vi "FPGA_main_simplified.vi"() -> ()   [LabVIEW 2024]
uses:
  <vilib>/Platform/TimedLoop/XDataNode/timing_clust.ctl
  <vilib>/Platform/TimedLoop/XDataNode/nitl_modes.ctl
  <vilib>/Platform/TimedLoop/XDataNode/wakeup.ctl
  <vilib>/LabVIEW Targets/FPGA/cRIO/shared/nicrio_ModuleControls/nicrio_cRIO-9775_ContinuousDataRates4ChansRing.ctl
  <vilib>/rvi/Emulation/niFpgaGetClockAttributes.vi
  <vilib>/rvi/Emulation/niFpgaSctlEmulationGetInTimedLoop.vi
  <vilib>/rvi/Emulation/niFpgaEmulationReportErrorSimple.vi
  <vilib>/rvi/Emulation/niFpgaProcessEmulError.vi
  <vilib>/rvi/Emulation/niFpgaCriticalErrorInLSC.vi
  <vilib>/rvi/eio/common/nirviEmuTemplateMethod_errors.vi
  <vilib>/rvi/eio/common/nirviEmuTemplatePropertySet_errors.vi
  <vilib>/eio/utilities/niEioResolveVilibRelativePath.vi
  <vilib>/rvi/interface/RandomDataEmulation/niFpgaRandomDataHandleErrors.vi
  <vilib>/platform/TimedLoop/XDataNode/XDataNode.xnode
  <vilib>/eio/EIONode/EIONode.xnode
  <vilib>/eio/EIOMethodNode/EIOMethodNode.xnode
  <vilib>/eio/EIOPropertyNode/EIOPropertyNode.xnode
  <vilib>/rvi/DataTransferAndStorage/Container/XNode/niFpgaContainer.xnode
  <vilib>/rvi/interface/RandomDataEmulation/nirviRandomDataFpgaReadWriteTemplate.vi
  <vilib>/Platform/TimedLoop/XDataNode/XDNodeRunTimeDep.lvlib
  <vilib>/rvi/eio/common/nirviEmuTemplatePropertyGet_errors.vi
  <vilib>/rvi/eio/common/nirviEmuTemplatePropertyGet_noerrors.vi
  <vilib>/rvi/eio/common/nirviEmuTemplatePropertySet_noerrors.vi
panel:
  out "FPGA routine\nrunning":bool
  in  "Pulse\nWidth":u32 caption="Pulse width(uSec)"
  in  "Pulse\nPeriod":u32 caption="Period(uSec)"
  in  "Stop Routine":bool
  in  "DIO3":bool
  in  "DIO2":bool
  in  "DIO1":bool
  in  "DIO0":bool
  out "Rebinned Counts":i32
  in  "Binning Time (ticks)":i32=1200000
  out "Counts":u8
  out "FPGA Error":errorcluster
  out "Finished":bool
  in  "Stop":bool
  out "Module Underflow":bool
  out "DMA FIFO Full":bool
  out "Actual Loop Period (ticks)":u32=40
  out "First Read":bool
  in  "Type Counter":enum16{"Falling Edge", "Rising Edge"}(ring)
  # "Photon counting. Single cycle time loop"
  # "User Control of digital output"
  # "Thresholding"
  # "Pulsing DIO 0 (Pulse width should be shorter than\n period)"
  # "Binning and streaming binned Total Count"
  # "Streaming Analog Input Data"
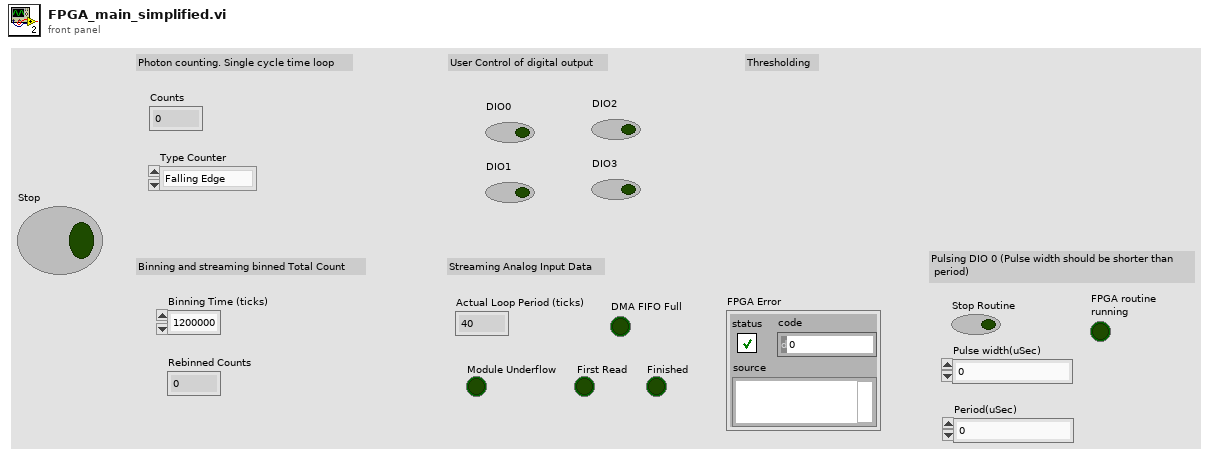
[diagram p1: front panel]
types:
  T1 = typedef "nicrio_cRIO-9775_ContinuousDataRates4ChansRing.ctl" = u16
  T2 = typedef "XDNodeRunTimeDep.lvlib/timing_clust.ctl" = cluster{"Expected End [f-1]":u64, "Actual End [f-1]":u64, "Finished Late? [f-1]":bool, "Expected End [i-1]":u64, "Actual End [i-1]":u64, "Finished Late? [i-1]":bool, "Expected Start [i]":u64, "Actual Start [i]":u64, "Expected Start [f]":u64, "Actual Start [f]":u64, "Source Name":string, "Structure Name":string, "Period":i64, "Deadline":i64, "Offset":i64, "Start":i64, "Priority":i32, "Timeout":i32, "Mode":T3, "Wakeup Reason":T4, "Error":errorcluster, "Source Type":string, "Secondary Source Type":string, "Global End Time":u64, "Global Start Time":u64, "Frame Duration":u64, "Iteration Duration":u64, "Assigned CPU":i32, "I/O Scan Engine Mode":u32}
  T3 = typedef "XDNodeRunTimeDep.lvlib/nitl_modes.ctl" = enum32{"No Change", "Process missed periods, maintain original phase", "Discard missed periods, maintain original phase", "Process missed periods, ignore original phase", "Discard missed periods, ignore original phase"}
  T4 = typedef "XDNodeRunTimeDep.lvlib/wakeup.ctl" = enum32{"Normal", "Aborted", "Asynchronous wakeup", "Timing source error", "Timed loop error", "Timeout"}
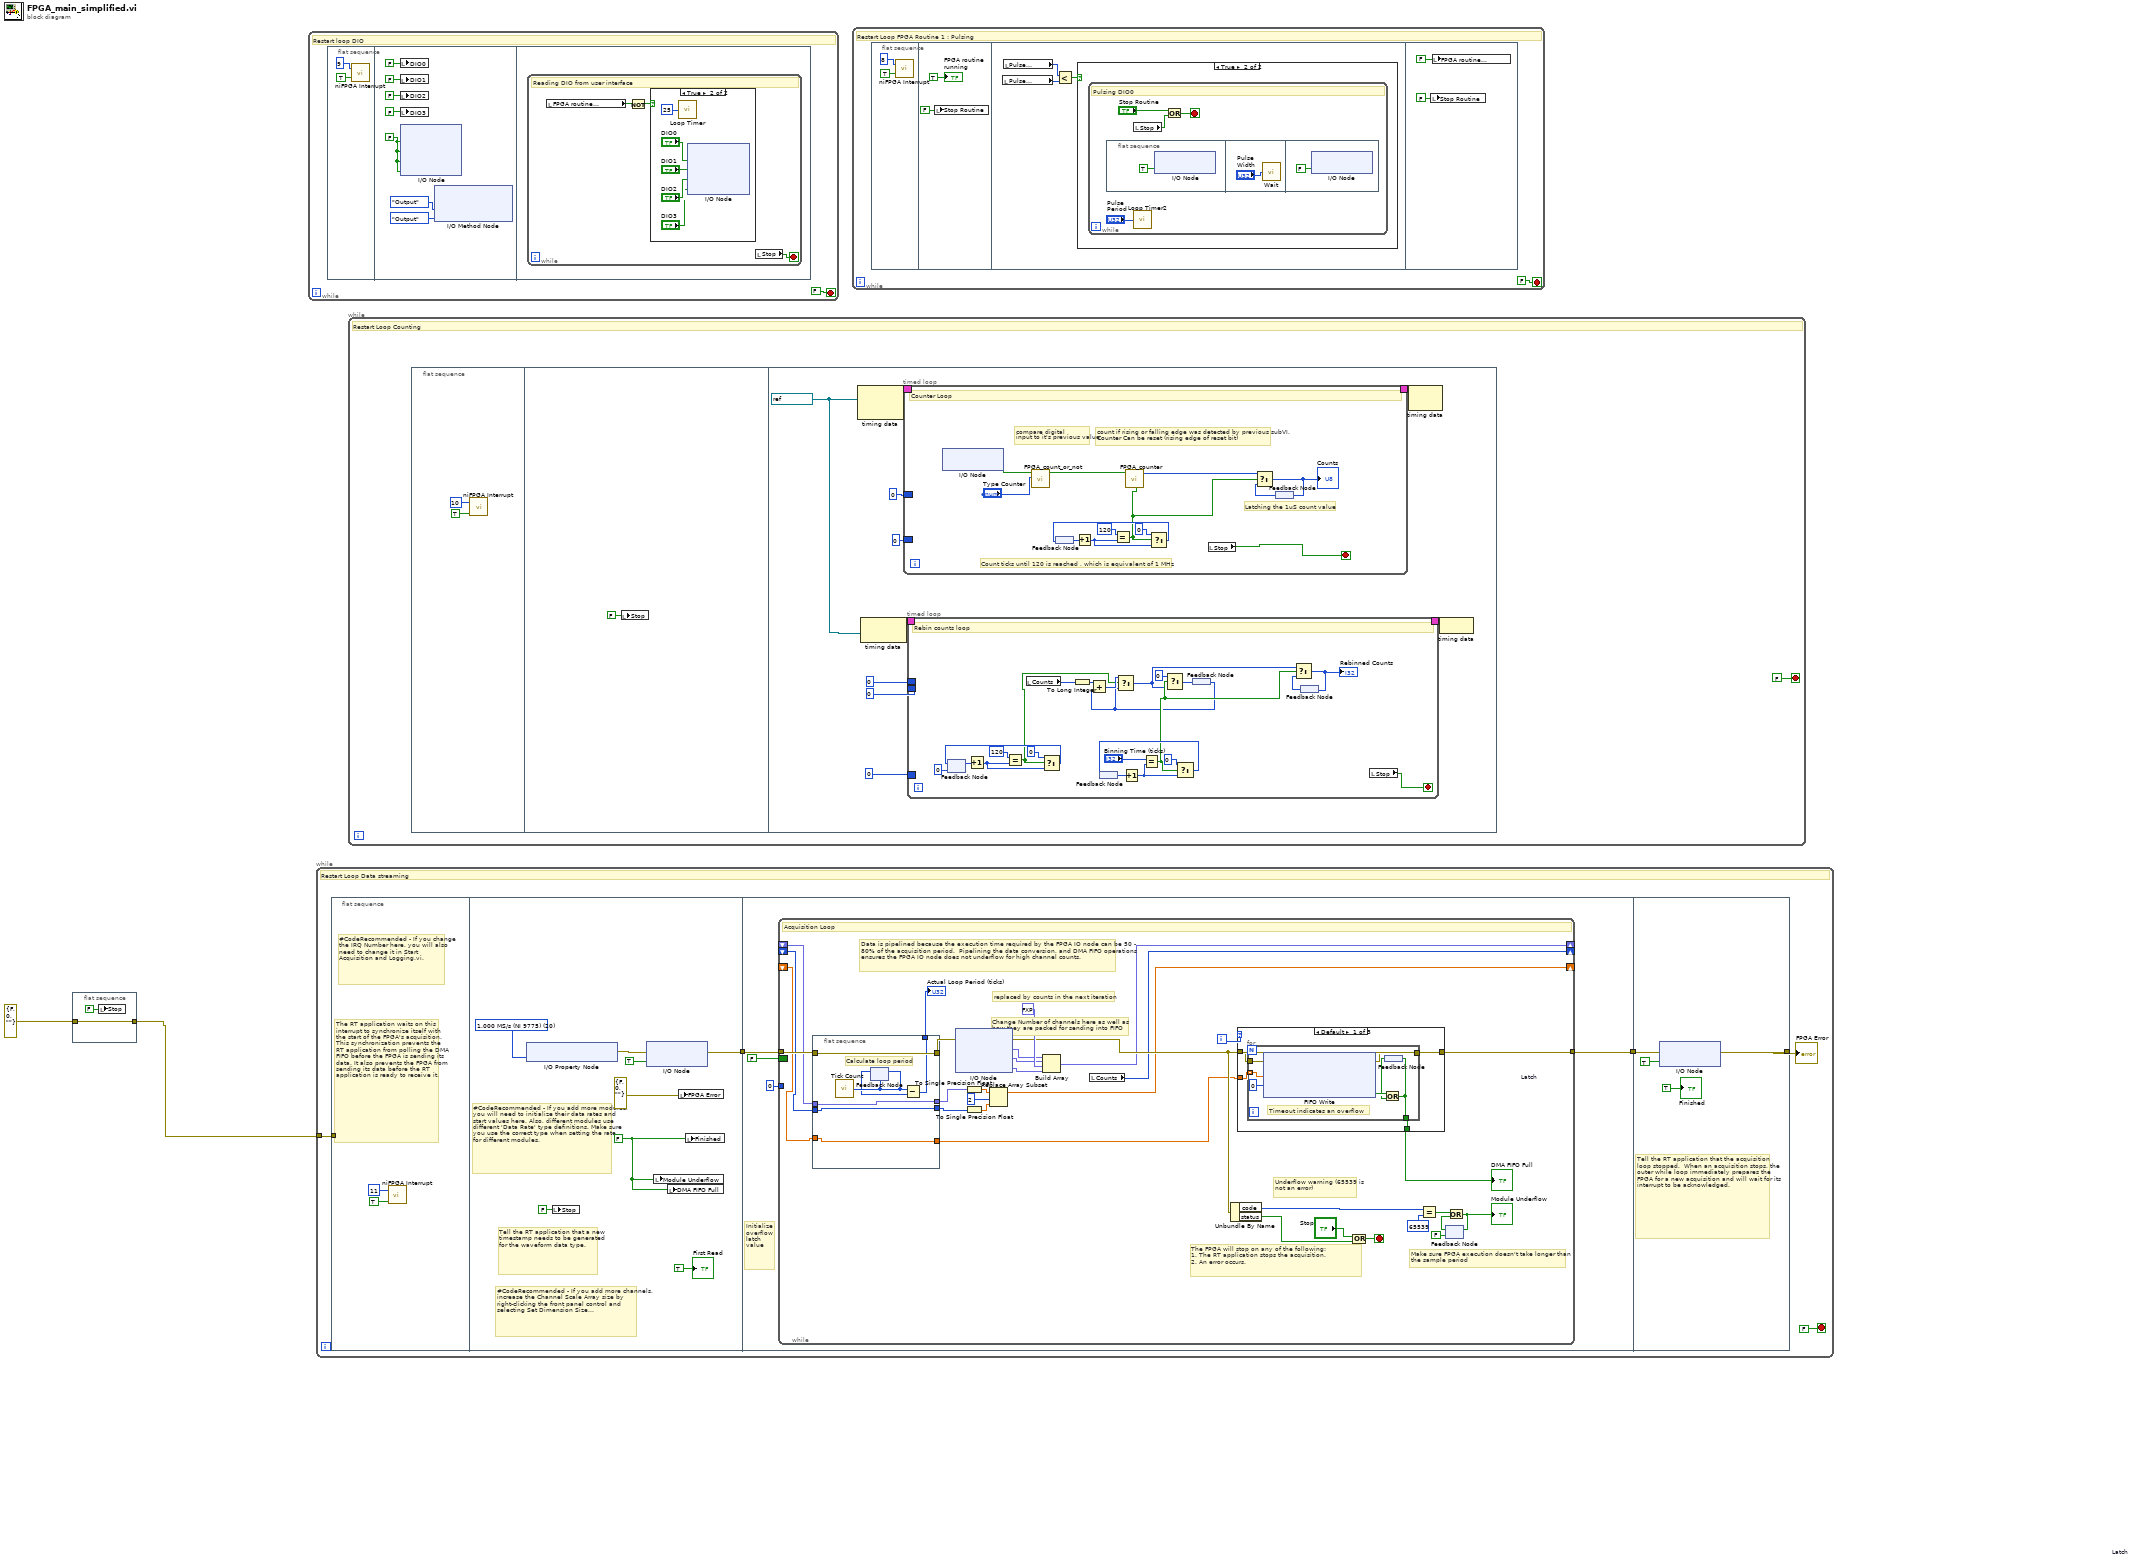
[diagram p0: block diagram]
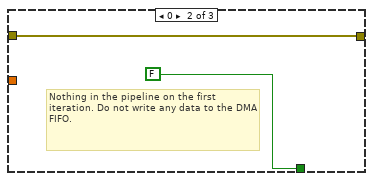
[diagram p4: hidden frame]
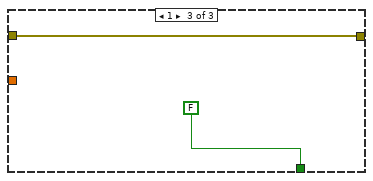
[diagram p5: hidden frame]
diagram:
  n1 = flat-sequence {
    tunnel: errorcluster {"status"=FALSE, "code"=0, "source"=""} ("Error") -> [w3]
    tunnel: [w3] -> w1
    frame #0 {
      n2 = local write "Stop"(FALSE ("stop")) -> ()
    }
  }
  n3 = while {
    stop <- FALSE stop-if-true
    # "Restart loop DIO"
    n4 = flat-sequence {
      frame #0 {
        n5 = call <vilib>:"niFPGA Interrupt.vi"("Wait Until Cleared (F)"=TRUE ("Wait Until Cleared"), "IRQ Number (0)"=u8 9 ("IRQ Number")) -> ()  [unwired: 1 in]
      }
      frame #1 {
        w10 = FALSE ("Mod3/DIO0")
        n6 = local write "DIO0"(FALSE ("DIO0")) -> ()
        n7 = local write "DIO1"(FALSE ("DIO1")) -> ()
        n8 = local write "DIO2"(FALSE ("DIO2")) -> ()
        n9 = local write "DIO3"(FALSE ("DIO3")) -> ()
        n10 = xnode "I/O Node"("Mod3/DIO0"=w10, "Mod3/DIO1"=w10, "Mod3/DIO2"=w10, "Mod3/DIO3"=w10) -> ()  [unwired: 4 in, 4 out]
        n11 = xnode "I/O Method Node"("DIO 7:4"=enum8{"No Change", "Input", "Output"}."Output", "DIO 3:0"=enum8{"No Change", "Input", "Output"}."Output") -> ()  [unwired: 1 in, 1 out]
      }
      frame #2 {
        n12 = while {
          stop <- w17 stop-if-true
          # "Reading DIO from user interface"
          n13 = local read "FPGA routine\nrunning"() -> (w16:bool)
          n14 = Not(x=w16) -> (.not. x?=w15:bool)
          n15 = case shown="True" w15 {
            frame False {
            }
            frame True {
              n16 = call "Loop Timer"("Count(mSec)"=u8 25) -> ()  [unwired: 1 out]
              n17 = xnode "I/O Node"("Mod3/DIO0"="DIO0", "Mod3/DIO1"="DIO1", "Mod3/DIO2"="DIO2", "Mod3/DIO3"="DIO3") -> ()  [unwired: 4 in, 4 out]
            }
          }
          n18 = local read "Stop"() -> (w17:bool)
        }
      }
    }
  }
  n19 = while {
    tunnel: w1 -> [w23]
    stop <- FALSE stop-if-true
    # "Restart Loop Data streaming"
    n20 = flat-sequence {
      tunnel: w23 -> [_]
      tunnel: [w37] -> w26
      tunnel: w26 -> [w39]
      tunnel: [w38] -> w25
      tunnel: w25 -> [w97]
      tunnel: [w96] -> w24
      frame #0 {
        # "#CodeRecommended - If you change the IRQ Number here, you will also need to change it in Start Acquisition and Logging.vi."
        # "The RT application waits on this interrupt to synchronize itself with the start of the FPGA's acquisition.  This synchronization prevents the RT application from polling the DMA FIFO before the FPGA is sending its data. It also prevents the FPGA from sending its data before the RT application is ready to receive it."
        n21 = call <vilib>:"niFPGA Interrupt.vi"("Wait Until Cleared (F)"=TRUE ("Wait Until Cleared"), "IRQ Number (0)"=u8 11 ("IRQ Number")) -> ()  [unwired: 1 in]
      }
      frame #1 {
        w31 = T1 20 items=["1.000 MS/s (NI 9775)"=20, "833.333 KS/s (NI 9775)"=24, "714.286 KS/s (NI 9775)"=28, "625.000 KS/s (NI 9775)"=32, "555.556 KS/s (NI 9775)"=36, "500.000 KS/s (NI 9775)"=40, "454.545 KS/s (NI 9775)"=44, "416.667 KS/s (NI 9775)"=48, "384.615 KS/s (NI 9775)"=52, "357.143 KS/s (NI 9775)"=56, "333.333 KS/s (NI 9775)"=60, "312.500 KS/s (NI 9775)"=64, "294.118 KS/s (NI 9775)"=68, "277.778 KS/s (NI 9775)"=72, "263.158 KS/s (NI 9775)"=76, "250.000 KS/s (NI 9775)"=80, "238.095 KS/s (NI 9775)"=84, "227.273 KS/s (NI 9775)"=88, "217.391 KS/s (NI 9775)"=92, "208.333 KS/s (NI 9775)"=96, "200.000 KS/s (NI 9775)"=100, "192.308 KS/s (NI 9775)"=104, "185.185 KS/s (NI 9775)"=108, "178.571 KS/s (NI 9775)"=112, "172.414 KS/s (NI 9775)"=116, "166.667 KS/s (NI 9775)"=120, "161.290 KS/s (NI 9775)"=124, "156.250 KS/s (NI 9775)"=128, "151.515 KS/s (NI 9775)"=132, "147.059 KS/s (NI 9775)"=136, "142.857 KS/s (NI 9775)"=140, "138.889 KS/s (NI 9775)"=144, "135.135 KS/s (NI 9775)"=148, "131.579 KS/s (NI 9775)"=152, "128.205 KS/s (NI 9775)"=156, "125.000 KS/s (NI 9775)"=160, "121.951 KS/s (NI 9775)"=164, "119.048 KS/s (NI 9775)"=168, "116.279 KS/s (NI 9775)"=172, "113.636 KS/s (NI 9775)"=176, "111.111 KS/s (NI 9775)"=180, "108.696 KS/s (NI 9775)"=184, "106.383 KS/s (NI 9775)"=188, "104.167 KS/s (NI 9775)"=192, "102.041 KS/s (NI 9775)"=196, "100.000 KS/s (NI 9775)"=200, "50.000 KS/s (NI 9775)"=400, "33.333 KS/s (NI 9775)"=600, "25.000 KS/s (NI 9775)"=800, "20.000 KS/s (NI 9775)"=1000, "16.667 KS/s (NI 9775)"=1200, "14.286 KS/s (NI 9775)"=1400, "12.500 KS/s (NI 9775)"=1600, "11.111 KS/s (NI 9775)"=1800, "10.000 KS/s (NI 9775)"=2000, "9.091 KS/s (NI 9775)"=2200, "8.333 KS/s (NI 9775)"=2400, "7.692 KS/s (NI 9775)"=2600, "7.143 KS/s (NI 9775)"=2800, "6.667 KS/s (NI 9775)"=3000, "6.250 KS/s (NI 9775)"=3200, "5.882 KS/s (NI 9775)"=3400, "5.556 KS/s (NI 9775)"=3600, "5.000 KS/s (NI 9775)"=4000, "4.762 KS/s (NI 9775)"=4200, "4.545 KS/s (NI 9775)"=4400, "4.348 KS/s (NI 9775)"=4600, "4.167 KS/s (NI 9775)"=4800, "4.000 KS/s (NI 9775)"=5000, "3.846 KS/s (NI 9775)"=5200, "3.571 KS/s (NI 9775)"=5600, "3.333 KS/s (NI 9775)"=6000, "3.125 KS/s (NI 9775)"=6400, "2.941 KS/s (NI 9775)"=6800, "2.778 KS/s (NI 9775)"=7200, "2.632 KS/s (NI 9775)"=7600, "2.500 KS/s (NI 9775)"=8000, "2.381 KS/s (NI 9775)"=8400, "2.273 KS/s (NI 9775)"=8800, "2.174 KS/s (NI 9775)"=9200, "2.083 KS/s (NI 9775)"=9600, "2.000 KS/s (NI 9775)"=10000, "1.923 KS/s (NI 9775)"=10400, "1.852 KS/s (NI 9775)"=10800, "1.786 KS/s (NI 9775)"=11200, "1.724 KS/s (NI 9775)"=11600, "1.667 KS/s (NI 9775)"=12000, "1.613 KS/s (NI 9775)"=12400, "1.563 KS/s (NI 9775)"=12800, "1.515 KS/s (NI 9775)"=13200, "1.471 KS/s (NI 9775)"=13600, "1.429 KS/s (NI 9775)"=14000, "1.389 KS/s (NI 9775)"=14400, "1.351 KS/s (NI 9775)"=14800, "1.316 KS/s (NI 9775)"=15200, "1.282 KS/s (NI 9775)"=15600, "1.250 KS/s (NI 9775)"=16000, "1.220 KS/s (NI 9775)"=16400, "1.190 KS/s (NI 9775)"=16800, "1.163 KS/s (NI 9775)"=17200, "1.136 KS/s (NI 9775)"=17600, "1.111 KS/s (NI 9775)"=18000, "1.087 KS/s (NI 9775)"=18400, "1.064 KS/s (NI 9775)"=18800, "1.042 KS/s (NI 9775)"=19200, "1.020 KS/s (NI 9775)"=19600, "1.000 KS/s (NI 9775)"=20000, "0.980 KS/s (NI 9775)"=20400, "0.962 KS/s (NI 9775)"=20800, "0.943 KS/s (NI 9775)"=21200, "0.926 KS/s (NI 9775)"=21600, "0.909 KS/s (NI 9775)"=22000, "0.893 KS/s (NI 9775)"=22400, "0.877 KS/s (NI 9775)"=22800, "0.862 KS/s (NI 9775)"=23200, "0.847 KS/s (NI 9775)"=23600, "0.833 KS/s (NI 9775)"=24000, "0.820 KS/s (NI 9775)"=24400, "0.806 KS/s (NI 9775)"=24800, "0.794 KS/s (NI 9775)"=25200, "0.781 KS/s (NI 9775)"=25600, "0.694 KS/s (NI 9775)"=28800, "0.625 KS/s (NI 9775)"=32000, "0.568 KS/s (NI 9775)"=35200, "0.521 KS/s (NI 9775)"=38400, "0.446 KS/s (NI 9775)"=44800, "0.391 KS/s (NI 9775)"=51200, "0.347 KS/s (NI 9775)"=57600, "0.313 KS/s (NI 9775)"=64000] ("Continuous Data Rate")
        w34 = FALSE ("Module Underflow")
        # "Tell the RT application that a new timestamp needs to be generated for the waveform data type."
        # "#CodeRecommended - If you add more channels, increase the Channel Scale Array size by right-clicking the front panel control and selecting Set Dimension Size..."
        # "#CodeRecommended - If you add more modules, you will need to initialize their data rates and start values here. Also, different modules use different 'Data Rate' type definitions. Make sure you use the correct type when setting the rate for different modules."
        n22 = xnode "I/O Property Node"("Continuous Data Rate"=w31) -> ("error out"=w33:errorcluster)  [unwired: 2 in, 1 out]
        n23 = local write "Stop"(FALSE ("Stop")) -> ()
        n24 = xnode "I/O Node"("error in"=w33, "Mod1/Start"=TRUE) -> ("error out"=w37:errorcluster)  [unwired: 1 in, 1 out]
        n25 = local write "Module Underflow"(w34) -> ()
        n26 = local write "DMA FIFO Full"(w34) -> ()
        n27 = local write "FPGA Error"(errorcluster {"status"=FALSE, "code"=0, "source"=""} ("FPGA Error")) -> ()
        n28 = local write "Finished"(w34) -> ()
        "First Read" <- TRUE ("First Read")
      }
      frame #2 {
        # "Initialize overflow latch value"
        n29 = while {
          tunnel: w39 -> [w68]
          tunnel: [w73] -> w38
          border: FALSE ("Overflow\nLatch") -> [_]
          tunnel: u8 0 ("Counts") -> [_]
          shift-right: [w56] -> _
          shift-left: _ -> [w55]
          shift-right: [w45] -> _
          shift-left: _ -> [w53]
          shift-right: [w51] -> _
          shift-left: _ -> [w50]
          i -> [w59]
          stop <- w72 stop-if-true
          # "replaced by counts in the next iteration"
          # "Data is pipelined because the execution time required by the FPGA IO node can be 50 - 80% of the acquisition period.  Pipelining the data conversion, and DMA FIFO operations ensures the FPGA IO node does not underflow for high channel counts."
          # "Change Number of channels here as well as \nhow they are packed for sending into FIFO"
          # "Underflow warning (65539 is not an error)"
          # "The FPGA will stop on any of the following:\n1. The RT application stops the acquisition.\n2. An error occurs."
          # "Make sure FPGA execution doesn't take longer than the sample period"
          # "Acquisition Loop"
          n30 = flat-sequence {
            tunnel: [w95] -> w67
            tunnel: w68 -> [w95]
            tunnel: [w92] -> w66
            tunnel: w55 -> [w91]
            tunnel: [w91] -> w54
            tunnel: w53 -> [w90]
            tunnel: [w90] -> w52
            tunnel: w50 -> [w89]
            tunnel: [w89] -> w49
            frame #0 {
              # "Calculate loop period"
              n31 = call "Tick Count"() -> ("Tick Count(Ticks)"=w94:u32)
              n32 = feedback-in #1(w94) -> ()
              n33 = feedback #1(w94) -> (w93:u32)
              n34 = Subtract(x=w94, y=w93) -> (x-y=w92:u32)
            }
          }
          n35 = xnode "I/O Node"("error in"=w67) -> ("error out"=w57:errorcluster, "Mod1/AI0"=w44:fxp<+/-,17,5>, "Mod1/AI1"=w43:fxp<+/-,17,5>, "Mod1/AI2"=w42:fxp<+/-,17,5>)  [unwired: 3 in, 3 out]
          n36 = To Single Precision Float(number=w54) -> (single precision float=w48:sgl[])
          n37 = To Single Precision Float(number=w49) -> (single precision float=w46:sgl)
          n38 = Replace Array Subset(array=w48, new element=w46, index=2) -> (w45:sgl[])
          n39 = Build Array(w44, w43, fxp<+/-,17,5> 0.0 ("element"), w42) -> (w56:fxp<+/-,17,5>[])
          n40 = local read "Counts"() -> (w51:u8)
          n41 = case shown="Default" w59 {
            tunnel: [w74 FALSE FALSE] -> w69
            tunnel: w52 -> [w77 _ _]
            tunnel: w57 -> [w76 w85 w87]
            tunnel: [w75 w85 w87] -> w73
            frame Default {
              n42 = for {
                tunnel: [w82] -> w74
                tunnel: w77 -> [w78] mode=indexing
                tunnel: w76 -> [w80]
                tunnel: [w79] -> w75
                # "Timeout indicates an overflow"
                n43 = xnode ("FIFO Write")("Element"=w78, "Timeout"=0, "error in (no error)"=w80) -> ("Timed Out?"=w84:bool, "error out"=w79:errorcluster)  [unwired: 1 in, 1 out]
                n44 = feedback #2 "Latch"() -> (w83:bool)
                n45 = Or(x=w84, y=w83) -> (x .or. y?=w82:bool)
                n46 = feedback-in #2(w82) -> ()
              }
            }
            frame 0 {
              # "Nothing in the pipeline on the first iteration. Do not write any data to the DMA FIFO."
            }
            frame 1 {
            }
          }
          "DMA FIFO Full" <- w69
          n47 = Unbundle By Name(w73) -> ("code"=w70:i32, "status"=w61:bool)
          n48 = Compound Arithmetic op=OR("Stop", w61) -> (w72:bool)
          n49 = Equal?(x=w70, y=65539) -> (x = y?=w63:bool)
          n50 = feedback #3 "Latch"(FALSE) -> (w65:bool)
          n51 = Or(x=w63, y=w65) -> (x .or. y?=w62:bool)
          "Module Underflow" <- w62
          n52 = feedback-in #3(w62) -> ()
          "Actual Loop Period (ticks)" <- w66
        }
      }
      frame #3 {
        # "Tell the RT application that the acquisition loop stopped.  When an acquisition stops, the outer while loop immediately prepares the FPGA for a new acquisition and will wait for its interrupt to be acknowledged."
        n53 = xnode "I/O Node"("error in"=w97, "Mod1/Stop"=TRUE) -> ("error out"=w96:errorcluster)  [unwired: 1 in, 1 out]
        "Finished" <- TRUE ("Finished")
      }
    }
    "FPGA Error" <- w24
  }
  n54 = while {
    stop <- FALSE stop-if-true
    # "Restart Loop Counting"
    n55 = flat-sequence {
      frame #0 {
        n56 = call <vilib>:"niFPGA Interrupt.vi"("Wait Until Cleared (F)"=TRUE ("Wait Until Cleared"), "IRQ Number (0)"=u8 10 ("IRQ Number")) -> ()  [unwired: 1 in]
      }
      frame #1 {
        n57 = local write "Stop"(FALSE ("Stop")) -> ()
      }
      frame #2 {
        w106 = refnum<k21> "120MHz" ("Source Name")
        n58 = node-c288(w106) -> (w113:T2)  [unwired: 1 in]
        n59 = node-c288(w106) -> (w109:T2)
        n60 = timed-loop {
          timing: w113 -> [_]
          timing-out: [_] -> w112
          border: u8 0 ("t") -> [_]
          border: u8 0 ("Total Count") -> [_]
          stop <- w143 stop-if-true
          # "Latching the 1uS count value"
          # "Count ticks until 120 is reached , which is equivalent of 1 MHz"
          # "count if rising or falling edge was detected by previous subVI. Counter Can be reset (rising edge of reset bit)"
          # "compare digital\ninput to it's previous value"
          # "Counter Loop"
          n61 = xnode "I/O Node"() -> ("Mod2/DIO0"=w154:bool)  [unwired: 1 in, 1 out]
          n62 = call "FPGA_count_or_not.vi"("Type Counter"="Type Counter", "Countable"=w154) -> ("Count or Not?"=w155:bool)  [unwired: 9 in]
          n63 = feedback #4() -> (w152:u8)
          n64 = Increment(x=w152) -> (x+1=w150:u8)
          n65 = Equal?(x=u8 120 ("y"), y=w150) -> (x = y?=w147:bool)
          n66 = call "FPGA_counter.vi"("Count or Not?"=w155, "Reset Photon Count"=w147) -> ("Total Count"=w146:u8)  [unwired: 8 in]
          n67 = Select(t=u8 0, s=w147, f=w150) -> (s? t:f=w148:u8)
          n68 = feedback-in #4(w148) -> ()
          n69 = local read "Stop"() -> (w143:bool)
          n70 = feedback #5() -> (w144:u8)
          n71 = Select(t=w146, s=w147, f=w144) -> (s? t:f=w145:u8)
          "Counts" <- w145
          n72 = feedback-in #5(w145) -> ()
        }
        n73 = timed-loop {
          timing: w109 -> [_]
          timing-out: [_] -> w108
          border: 0 ("Counts") -> [_]
          border: 0 ("t") -> [_]
          border: 0 -> [_]
          stop <- w126 stop-if-true
          # "Rebin counts loop"
          n74 = feedback #6(u8 0 ("t")) -> (w123:u8)
          n75 = Increment(x=w123) -> (x+1=w121:u8)
          n76 = Equal?(x=u8 120 ("y"), y=w121) -> (x = y?=w116:bool)
          n77 = local read "Counts"() -> (w125:u8)
          n78 = Select(t=u8 0, s=w116, f=w121) -> (s? t:f=w119:u8)
          n79 = feedback-in #6(w119) -> ()
          n80 = To Long Integer(number=w125) -> (32bit integer=w124:i32)
          n81 = feedback #7() -> (w133:i32)
          n82 = Increment(x=w133) -> (x+1=w134:i32)
          n83 = Equal?(x="Binning Time (ticks)", y=w134) -> (x = y?=w129:bool)
          n84 = Select(t=0, s=w129, f=w134) -> (s? t:f=w136:i32)
          n85 = feedback-in #7(w136) -> ()
          n86 = feedback #8() -> (w117:i32)
          n87 = Add(x=w124, y=w117) -> (x+y=w118:i32)
          n88 = Select(t=w118, s=w116, f=w117) -> (s? t:f=w114:i32)
          n89 = Select(t=0, s=w129, f=w114) -> (s? t:f=w128:i32)
          n90 = feedback-in #8(w128) -> ()
          n91 = feedback #9() -> (w130:i32)
          n92 = Select(t=w114, s=w129, f=w130) -> (s? t:f=w131:i32)
          "Rebinned Counts" <- w131
          n93 = feedback-in #9(w131) -> ()
          n94 = local read "Stop"() -> (w126:bool)
        }
        n95 = node-c288(w112) -> ()  [unwired: 1 out]
        n96 = node-c288(w108) -> ()
      }
    }
  }
  n97 = while {
    stop <- FALSE stop-if-true
    # "Restart Loop FPGA Routine 1 : Pulsing"
    n98 = flat-sequence {
      frame #0 {
        n99 = call <vilib>:"niFPGA Interrupt.vi"("Wait Until Cleared (F)"=TRUE ("Wait Until Cleared"), "IRQ Number (0)"=u8 8 ("IRQ Number")) -> ()  [unwired: 1 in]
      }
      frame #1 {
        n100 = local write "Stop Routine"(FALSE ("Stop Routine")) -> ()
        "FPGA routine\nrunning" <- TRUE
      }
      frame #2 {
        n101 = local read "Pulse\nPeriod"() -> (w168:u32)
        n102 = local read "Pulse\nWidth"() -> (w169:u32)
        n103 = Less?(x=w169, y=w168) -> (x < y?=w167:bool)
        n104 = case shown="True" w167 {
          frame False {
          }
          frame True {
            n105 = while {
              stop <- w172 stop-if-true
              # "Pulsing DIO0"
              n106 = flat-sequence {
                frame #0 {
                  n107 = xnode "I/O Node"("Mod3/DIO0"=TRUE) -> ()  [unwired: 1 in, 1 out]
                }
                frame #1 {
                  n108 = call "Wait"("Count(uSec)"="Pulse\nWidth") -> ()  [unwired: 1 out]
                }
                frame #2 {
                  n109 = xnode "I/O Node"("Mod3/DIO0"=FALSE) -> ()  [unwired: 1 in, 1 out]
                }
              }
              n110 = local read "Stop"() -> (w173:bool)
              n111 = call "Loop Timer2"("Count(uSec)"="Pulse\nPeriod") -> ()  [unwired: 1 out]
              n112 = Or(x="Stop Routine", y=w173) -> (x .or. y?=w172:bool)
            }
          }
        }
      }
      frame #3 {
        n113 = local write "Stop Routine"(FALSE ("Stop Routine")) -> ()
        n114 = local write "FPGA routine\nrunning"(FALSE ("FPGA routine\nrunning")) -> ()
      }
    }
  }
